vi "visibling and invisibling items.vi"() -> ()   [LabVIEW 2018]
panel:
  in  "String":string
  in  "stop 2":bool
  in  "stop 2":bool
  in  "VISIBLE":bool
  in  "Boolean 2":bool
  in  "stop":bool
  out "Visible":bool
  in  "Boolean":bool
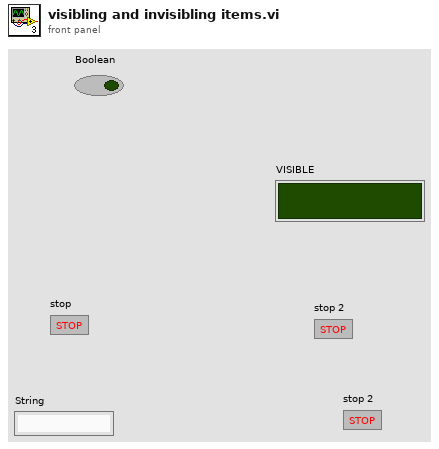
[diagram p1: front panel]
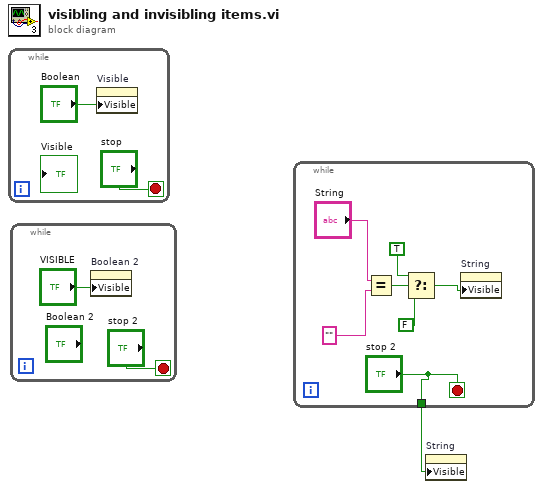
[diagram p0: block diagram]
diagram:
  n1 = while {
    stop <- "stop" stop-if-true
    n2 = property on="Visible" class="Bool (strict)"("Visible"="Boolean") -> ()  [unwired: 2 in, 2 out]
  }
  n3 = while {
    stop <- "stop 2" stop-if-true
    n4 = property on="Boolean 2" class="Bool (strict)"("Visible"="VISIBLE") -> ()  [unwired: 2 in, 2 out]
  }
  n5 = while {
    tunnel: ["stop 2"] -> w1
    stop <- "stop 2" stop-if-true
    n6 = Equal?(x="String", y="") -> (x = y?=w11:bool)
    n7 = Select(t=TRUE ("Boolean"), s=w11, f=FALSE ("Boolean")) -> (s? t:f=w7:bool)
    n8 = property on="String" class="Str"("Visible"=w7) -> ()  [unwired: 2 in, 2 out]
  }
  n9 = property on="String" class="Str"("Visible"=w1) -> ()  [unwired: 2 in, 2 out]
